vi "RefNums.vi"() -> ()   [LabVIEW 2013, in "ProjectHandler.lvlib"]
uses:
  ProjectHandler.lvlib
panel:
  in  "RefNums":T1
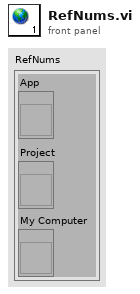
[diagram p1: front panel]
types:
  T1 = cluster{"App":refnum<vi>, "Project":refnum<vi>, "My Computer":refnum<vi>}
diagram:
